vi "ABB cool curve report.vi"(10 "Report in":string, 11 "Heat run #":i32) -> (2 "Report out":string)   [LabVIEW 2017]
uses:
  ABB global.vi
panel:
  out "Motor Type":string
  out "Rotor Cooling curve":T1(graph)
  out "Stator cooling Curve":T1(graph)
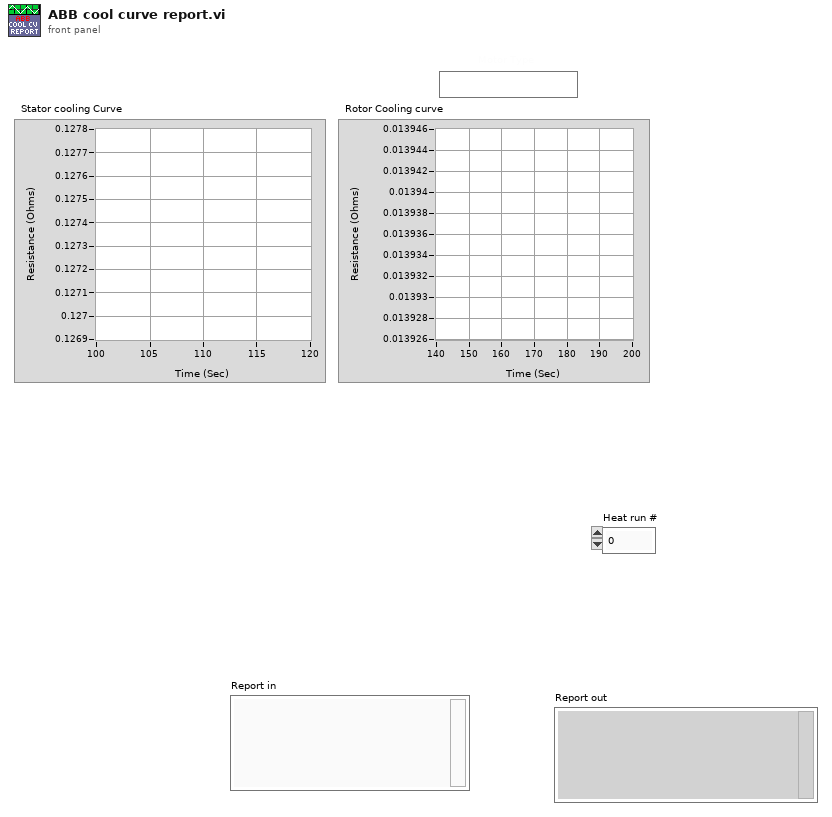
[diagram p1: front panel]
types:
  T1 = cluster{"No load test results":dbl[], "No load test results":dbl[]}
  T2 = cluster{"Stator R":dbl, "Stator dT":dbl, "Rotor R":dbl, "Rotor dT":dbl, "Stator Cooling curve":dbl[][], "Rotor Cooling curve":dbl[][], "Select Resistance":enum16{"Fitted zero Res.", "Selected Res.", "Entered Res."}}[]
  T3 = cluster{"Stator R":dbl, "Stator dT":dbl, "Rotor R":dbl, "Rotor dT":dbl, "Stator Cooling curve":dbl[][], "Rotor Cooling curve":dbl[][], "Select Resistance":enum16{"Fitted zero Res.", "Selected Res.", "Entered Res."}}
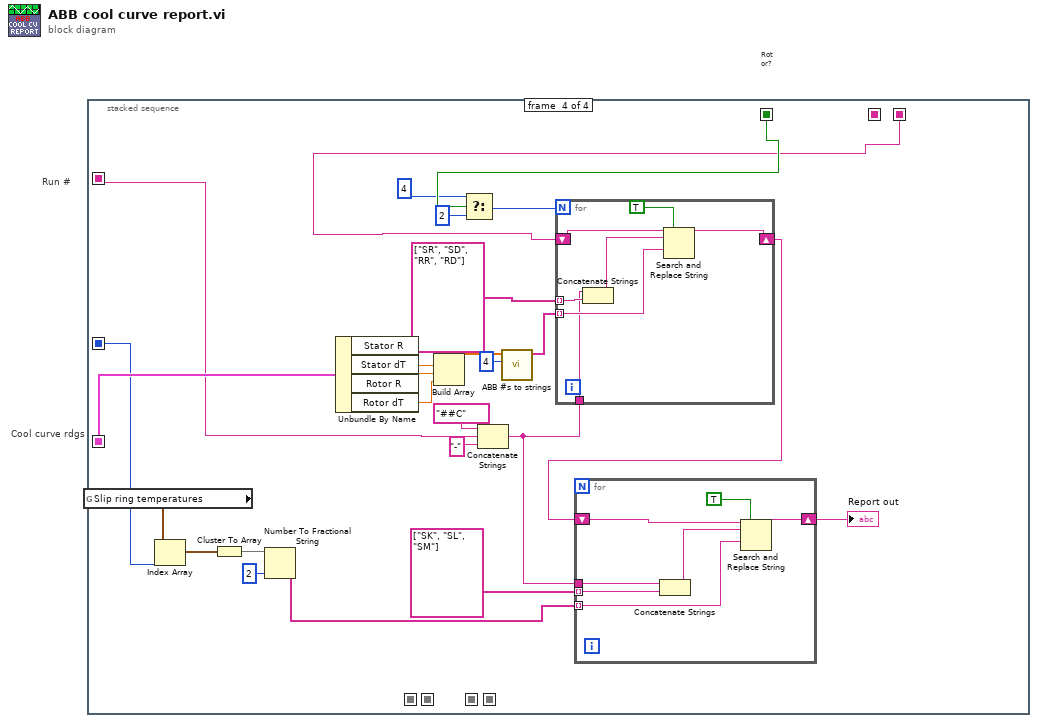
[diagram p0: block diagram]
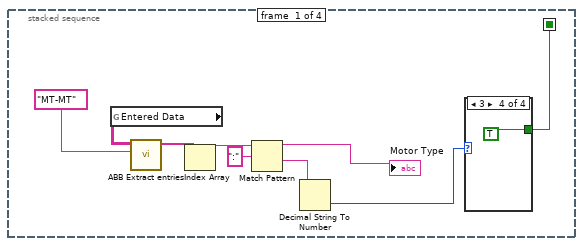
[diagram p2: hidden frame]
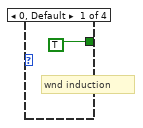
[diagram p3: hidden frame]
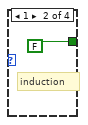
[diagram p4: hidden frame]
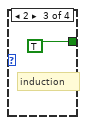
[diagram p5: hidden frame]
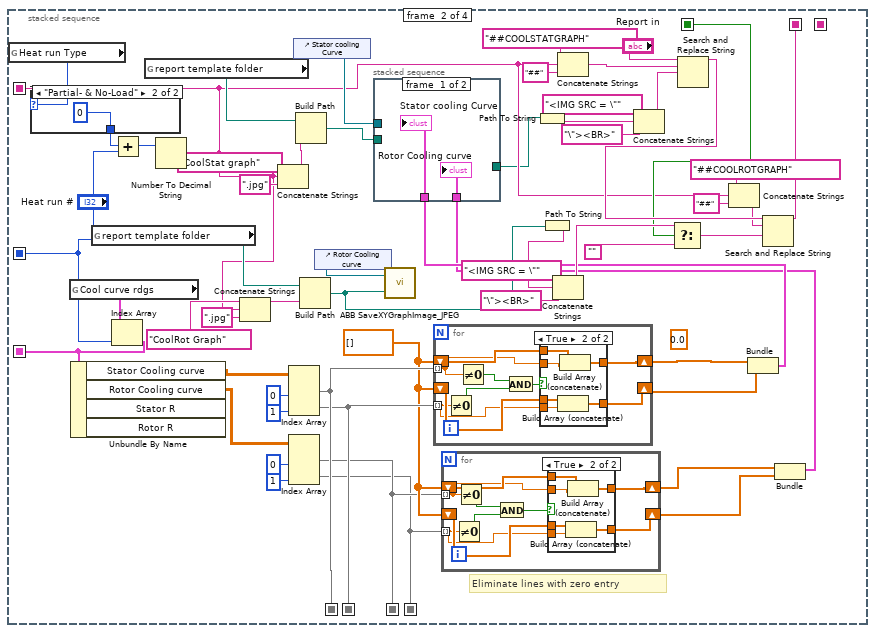
[diagram p6: hidden frame]
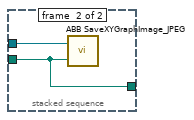
[diagram p7: hidden frame]
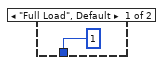
[diagram p8: hidden frame]
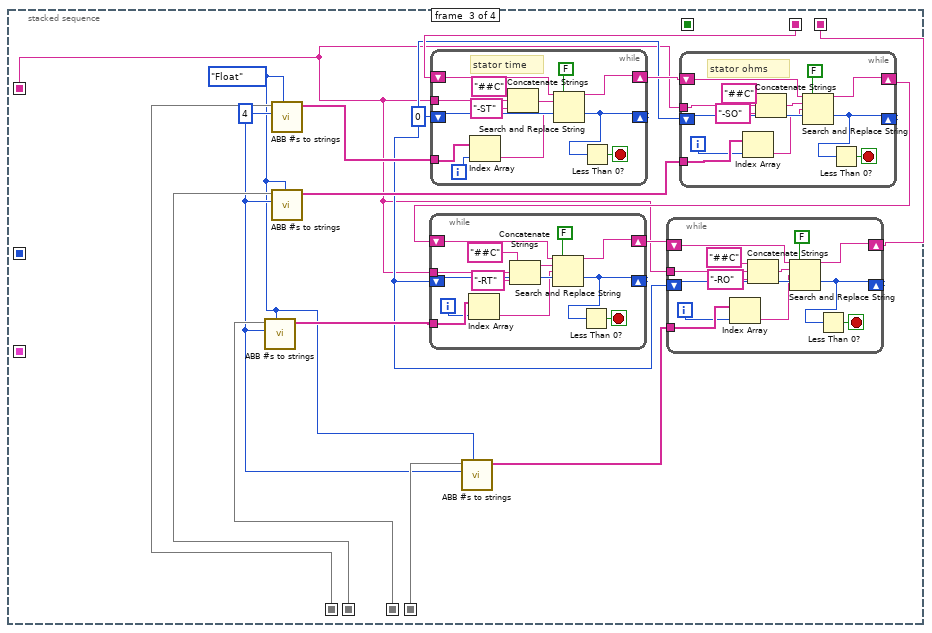
[diagram p11: hidden frame]
diagram:
  # "Cool curve rdgs"
  # "Run #"
  # "Rotor?"
  n1 = stacked-sequence {
    seq-local: [_ w55 _ _] -> [_ _ w126 _]
    seq-local: [_ w49 _ _] -> [_ _ w121 _]
    seq-local: [_ w50 _ _] -> [_ _ w122 _]
    seq-local: [_ w47 _ _] -> [_ _ w119 _]
    seq-local: [_ w46 _ _] -> [_ _ w117 _]
    seq-local: [_ _ w112 _] -> [_ _ _ w205]
    seq-local: [w1 _ _ _] -> [_ w41 _ w206]
    seq-local: [_ w26 _ _] -> [_ _ w111 w190]
    seq-local: [_ w24 _ _] -> [_ _ _ w191]
    seq-local: [_ "Heat run #" _ _] -> [_ _ _ w185]
    frame #0 {
      n2 = global read "ABB global.vi" "Entered Data"() -> (w9:string[][])
      n3 = call "ABB Extract entries.vi"("Entry ID"="MT-MT", "Entry table in"=w9) -> ("Selected Entries"=w4:string[])  [unwired: 9 in]
      n4 = Index Array(array=w4) -> (element=w3:string)  [unwired: 1 in]
      n5 = Match Pattern(string=w3, regular expression=":") -> (before substring=→"Motor Type":string, after substring=w6:string)  [unwired: 1 in, 2 out]
      n6 = Decimal String To Number(string=w6) -> (number=w2:i32)  [unwired: 2 in, 1 out]
      n7 = case shown="3" w2 {
        tunnel: [TRUE FALSE TRUE TRUE] -> w1
        frame 0, Default {
          # "wnd induction"
        }
        frame 1 {
          # "induction"
        }
        frame 2 {
          # "induction"
        }
        frame 3 {
        }
      }
    }
    frame #1 {
      (unwired) 0.0
      w48 = dbl[] []
      # "Eliminate lines with zero entry"
      n8 = global read "ABB global.vi" "Heat run Type"() -> (w23:enum16{"Full Load", "Partial- & No-Load"})
      n9 = case shown="\"Partial- & No-Load\"" w23 {
        tunnel: [1 0] -> w22
        frame "Full Load", Default {
        }
        frame "Partial- & No-Load" {
        }
      }
      n10 = global read "ABB global.vi" "Cool curve rdgs"() -> (w39:T2)
      n11 = global read "ABB global.vi" "report template folder"() -> (w62:path)
      n12 = Index Array(array=w39, index="Heat run #") -> (element=w24:T3)
      n13 = Unbundle By Name(w24) -> ("Stator Cooling curve"=w45:dbl[][], "Rotor Cooling curve"=w44:dbl[][])  [unwired: 2 out]
      n14 = Add(x=w22, y="Heat run #") -> (x+y=w38:i32)
      n15 = global read "ABB global.vi" "report template folder"() -> (w64:path)
      n16 = Number To Decimal String(number=w38) -> (decimal integer string=w26:string)  [unwired: 1 in]
      n17 = Concatenate Strings("CoolRot Graph" ("name or relative path"), w26, ".jpg" ("string")) -> (w25:string)
      n18 = Concatenate Strings("CoolStat graph" ("name or relative path"), w26, ".jpg" ("string")) -> (w29:string)
      n19 = Index Array(array=w45, index (col) #1=0 ("disabled index (col)"), index (col) #2=1 ("index (col)")) -> (element #1=w50:dbl[], element #2=w49:dbl[])  [unwired: 2 in]
      n20 = Index Array(array=w44, index (col) #1=0 ("disabled index (col)"), index (col) #2=1 ("index (col)")) -> (element #1=w47:dbl[], element #2=w46:dbl[])  [unwired: 2 in]
      n21 = control-ref of="Stator cooling Curve"() -> (w63:refnum<vi>)
      n22 = Build Path(base path=w64, name or relative path=w29) -> (appended path=w67:path)
      n23 = Build Path(base path=w62, name or relative path=w25) -> (appended path=w60:path)
      n24 = control-ref of="Rotor Cooling curve"() -> (w57:refnum<vi>)
      n25 = call "ABB SaveXYGraphImage_JPEG.vi"("Path"=w60, "COntrolReference"=w57) -> ()  [unwired: 2 in]
      n26 = for {
        shift-right: [w99] -> w18
        shift-left: w48 -> [w100]
        shift-right: [w96] -> w16
        shift-left: w48 -> [w98]
        tunnel: w50 -> [w94] mode=indexing
        tunnel: w49 -> [w97] mode=indexing
        n27 = Not Equal To 0?(x=w97) -> (x != 0?=w102:bool)
        n28 = Not Equal To 0?(x=w94) -> (x != 0?=w95:bool)
        n29 = And(x=w95, y=w102) -> (x .and. y?=w101:bool)
        n30 = case shown="True" w101 {
          tunnel: w100 -> [w104 w110]
          tunnel: w94 -> [_ w109]
          tunnel: [w104 w108] -> w99
          tunnel: w98 -> [w103 w107]
          tunnel: w97 -> [_ w106]
          tunnel: [w103 w105] -> w96
          frame False {
          }
          frame True {
            n31 = Build Array (concatenate)(w107, w106) -> (w105:dbl[])
            n32 = Build Array (concatenate)(w110, w109) -> (w108:dbl[])
          }
        }
      }
      n33 = for {
        shift-right: [w82] -> w17
        shift-left: w48 -> [w83]
        shift-right: [w79] -> w15
        shift-left: w48 -> [w81]
        tunnel: w47 -> [w77] mode=indexing
        tunnel: w46 -> [w80] mode=indexing
        n34 = Not Equal To 0?(x=w80) -> (x != 0?=w85:bool)
        n35 = Not Equal To 0?(x=w77) -> (x != 0?=w78:bool)
        n36 = And(x=w78, y=w85) -> (x .and. y?=w84:bool)
        n37 = case shown="True" w84 {
          tunnel: w83 -> [w87 w93]
          tunnel: w77 -> [_ w92]
          tunnel: [w87 w91] -> w82
          tunnel: w81 -> [w86 w90]
          tunnel: w80 -> [_ w89]
          tunnel: [w86 w88] -> w79
          frame False {
          }
          frame True {
            n38 = Build Array (concatenate)(w90, w89) -> (w88:dbl[])
            n39 = Build Array (concatenate)(w93, w92) -> (w91:dbl[])
          }
        }
      }
      n40 = Path To String(path=w60) -> (string=w61:string)
      n41 = Concatenate Strings("<IMG SRC = \"", w61, "\"><BR>" ("string")) -> (w42:string)
      n42 = Concatenate Strings("##COOLSTATGRAPH", w26, "##" ("string")) -> (w35:string)
      n43 = Select(t=w42, s=w41, f="") -> (s? t:f=w43:string)
      n44 = Concatenate Strings("##COOLROTGRAPH", w26, "##" ("string")) -> (w32:string)
      n45 = Bundle(w18, w16) -> (w20:cluster{dbl[], dbl[]})  [unwired: 1 in]
      n46 = Bundle(w17, w15) -> (w19:cluster{dbl[], dbl[]})  [unwired: 1 in]
      n47 = stacked-sequence {
        tunnel: w67 -> [_ w73]
        tunnel: w63 -> [_ w74]
        tunnel: [_ w73] -> w21
        tunnel: w20 -> [w72 _]
        tunnel: w19 -> [w71 _]
        frame #0 {
          "Stator cooling Curve" <- w72
          "Rotor Cooling curve" <- w71
        }
        frame #1 {
          n48 = call "ABB SaveXYGraphImage_JPEG.vi"("Path"=w73, "COntrolReference"=w74) -> ()  [unwired: 2 in]
        }
      }
      n49 = Path To String(path=w21) -> (string=w66:string)
      n50 = Concatenate Strings("<IMG SRC = \"", w66, "\"><BR>" ("string")) -> (w68:string)
      n51 = Search and Replace String(input string="Report in", search string=w35, replace string=w68) -> (result string=w56:string)  [unwired: 5 in, 3 out]
      n52 = Search and Replace String(input string=w56, search string=w32, replace string=w43) -> (result string=w55:string)  [unwired: 5 in, 3 out]
    }
    frame #2 {
      w114 = enum16{"Float", "Relative time HH:MM"}."Float" ("# type")
      w115 = 4 ("Precision")
      w113 = 0
      n53 = call "ABB #s to strings.vi"("# type"=w114, "Precision"=w115, "Numbers in"=w119) -> ("Strings out"=w118:string[])  [unwired: 8 in]
      n54 = call "ABB #s to strings.vi"("# type"=w114, "Precision"=w115, "Numbers in"=w122) -> ("Strings out"=w123:string[])  [unwired: 8 in]
      n55 = call "ABB #s to strings.vi"("# type"=w114, "Precision"=w115, "Numbers in"=w121) -> ("Strings out"=w120:string[])  [unwired: 8 in]
      n56 = while {
        shift-right: [w178] -> w127
        shift-left: w126 -> [w179]
        tunnel: w123 -> [w173]
        shift-right: [w174] -> _
        shift-left: w113 -> [w177]
        tunnel: w111 -> [w169]
        i -> [w172]
        stop <- w175 stop-if-true
        # "stator time"
        n57 = Index Array(array=w173, index=w172) -> (element=w171:string)
        n58 = Concatenate Strings("##C" ("search string"), w169, "-ST" ("string")) -> (w168:string)
        n59 = Search and Replace String(replace all?=FALSE ("replace all? (F)"), input string=w179, search string=w168, replace string=w171, offset=w177) -> (result string=w178:string, offset past replacement=w174:i32)  [unwired: 3 in, 2 out]
        n60 = Less Than 0?(x=w174) -> (x < 0?=w175:bool)
      }
      n61 = call "ABB #s to strings.vi"("# type"=w114, "Precision"=w115, "Numbers in"=w117) -> ("Strings out"=w116:string[])  [unwired: 8 in]
      n62 = while {
        shift-right: [w165] -> w125
        shift-left: w127 -> [w166]
        tunnel: w120 -> [w160]
        shift-right: [w161] -> _
        shift-left: w113 -> [w164]
        tunnel: w111 -> [w155]
        i -> [w159]
        stop <- w162 stop-if-true
        # "stator ohms"
        n63 = Index Array(array=w160, index=w159) -> (element=w158:string)
        n64 = Concatenate Strings("##C" ("search string"), w155, "-SO" ("string")) -> (w157:string)
        n65 = Search and Replace String(replace all?=FALSE ("replace all? (F)"), input string=w166, search string=w157, replace string=w158, offset=w164) -> (result string=w165:string, offset past replacement=w161:i32)  [unwired: 3 in, 2 out]
        n66 = Less Than 0?(x=w161) -> (x < 0?=w162:bool)
      }
      n67 = while {
        shift-right: [w152] -> w124
        shift-left: w125 -> [w153]
        tunnel: w118 -> [w147]
        shift-right: [w148] -> _
        shift-left: w113 -> [w151]
        tunnel: w111 -> [w142]
        i -> [w146]
        stop <- w149 stop-if-true
        n68 = Index Array(array=w147, index=w146) -> (element=w145:string)
        n69 = Concatenate Strings("##C" ("search string"), w142, "-RT" ("string")) -> (w143:string)
        n70 = Search and Replace String(replace all?=FALSE ("replace all? (F)"), input string=w153, search string=w143, replace string=w145, offset=w151) -> (result string=w152:string, offset past replacement=w148:i32)  [unwired: 3 in, 2 out]
        n71 = Less Than 0?(x=w148) -> (x < 0?=w149:bool)
      }
      n72 = while {
        shift-right: [w139] -> w112
        shift-left: w124 -> [w140]
        tunnel: w116 -> [w134]
        shift-right: [w135] -> _
        shift-left: w113 -> [w138]
        tunnel: w111 -> [w130]
        i -> [w133]
        stop <- w136 stop-if-true
        n73 = Index Array(array=w134, index=w133) -> (element=w132:string)
        n74 = Concatenate Strings("##C" ("search string"), w130, "-RO" ("string")) -> (w131:string)
        n75 = Search and Replace String(replace all?=FALSE ("replace all? (F)"), input string=w140, search string=w131, replace string=w132, offset=w138) -> (result string=w139:string, offset past replacement=w135:i32)  [unwired: 3 in, 2 out]
        n76 = Less Than 0?(x=w135) -> (x < 0?=w136:bool)
      }
    }
    frame #3 {
      n77 = global read "ABB global.vi" "Slip ring temperatures"() -> (w186:cluster{"K":dbl, "L":dbl, "M ":dbl}[])
      n78 = Index Array(array=w186, index=w185) -> (element=w184:cluster{"K":dbl, "L":dbl, "M ":dbl})
      n79 = Cluster To Array(cluster=w184) -> (array=w183:dbl[])
      n80 = Number To Fractional String(number=w183, precision (6)=i16 2) -> (F-format string=w181:string[])  [unwired: 2 in]
      n81 = Unbundle By Name(w191) -> ("Stator R"=w203:dbl, "Stator dT"=w202:dbl, "Rotor R"=w201:dbl, "Rotor dT"=w200:dbl)
      n82 = Build Array(w203, w202, w201, w200) -> (w199:dbl[])
      n83 = Select(t=4, s=w206, f=2) -> (s? t:f=w194:i32)
      n84 = Concatenate Strings("##C", w190, "-") -> (w187:string)
      n85 = call "ABB #s to strings.vi"("Precision"=4, "Numbers in"=w199) -> ("Strings out"=w197:string[])  [unwired: 9 in]
      n86 = for {
        N: w194 -> [_]
        shift-right: [w219] -> w189
        shift-left: w205 -> [w220]
        tunnel: string[] ["SR", "SD", "RR", "RD"] -> [w216] mode=indexing
        tunnel: w197 -> [w217] mode=indexing
        tunnel: w187 -> [w215]
        n87 = Concatenate Strings(w215, w216) -> (w214:string)
        n88 = Search and Replace String(replace all?=TRUE ("replace all? (F)"), input string=w220, search string=w214, replace string=w217) -> (result string=w219:string)  [unwired: 4 in, 3 out]
      }
      n89 = for {
        shift-right: [w211] -> w188
        shift-left: w189 -> [w210]
        tunnel: w187 -> [w209]
        tunnel: w181 -> [w208] mode=indexing
        tunnel: string[] ["SK", "SL", "SM"] -> [w207] mode=indexing
        n90 = Concatenate Strings(w209, w207) -> (w213:string)
        n91 = Search and Replace String(replace all?=TRUE ("replace all? (F)"), input string=w210, search string=w213, replace string=w208) -> (result string=w211:string)  [unwired: 4 in, 3 out]
      }
      "Report out" <- w188
    }
  }
